vi "daqio_Upload_File.vi"(8 "error in (no error)":errorcluster, 10 "File to upload":T1={"File Type"="image", "label (File Name by default)"="", "File to be uploaded"=path ""}, 11 "daq.io type in":T2={"daq.io ref"=refnum, "daq.io API Base"="http://dashboard.daq.io/api/v1", "Device Key"="", "Account ID"="", "online"=TRUE, "SSL"=TRUE}) -> (0 "error out":errorcluster, 2 "asset ID":string, 3 "daq.io type out":T2={"daq.io ref"=refnum, "daq.io API Base"="http://dashboard.daq.io/api/v1", "Device Key"="", "Account ID"="", "online"=TRUE, "SSL"=TRUE})   [LabVIEW 2013, in "daqio minimal.lvlib"]
doc: "This VI uploads a new user file. It can be any file type. However, images and CSV files will be treated specially on daq.io, therefore make sure to select the correct file type, if you want features like the image preview to work. For PDF files, please select binary. \nThe VI will return the unique file ID that can be used to retrieve the file later and link it to a device."
uses:
  daqio minimal.lvlib
  _typedefs/daqio-Type.ctl
  <vilib>/httpClient/ClientHandle.ctl
  _typedefs/daqio-File.ctl
  _typedefs/daqio-File-Post.ctl
  <vilib>/httpClient/MultipartData.ctl
  _typedefs/daqio-Credentials-FGV.ctl
  <vilib>/Easy HTTP Client/Easy HTTP.lvlib
  <vilib>/httpClient/LabVIEWHTTPClient.lvlib
panel:
  out "JSON string":string
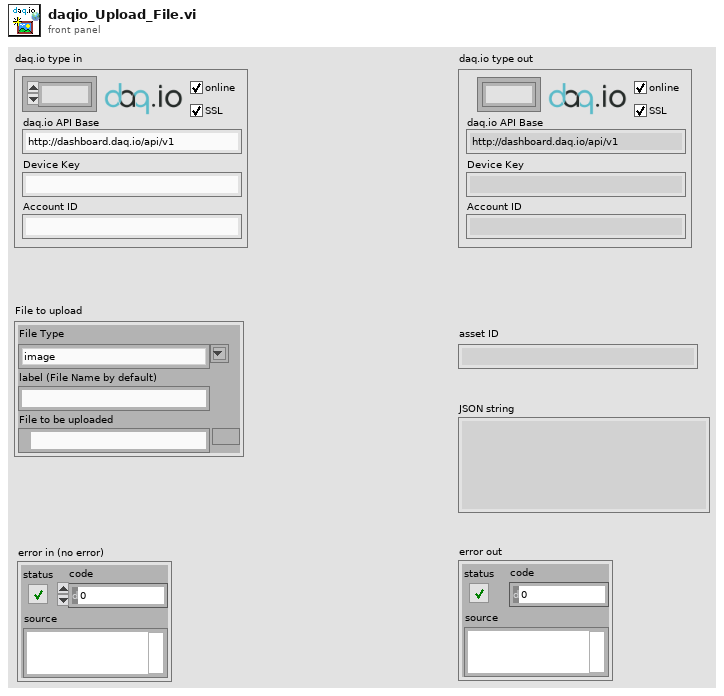
[diagram p1: front panel]
types:
  T1 = cluster{"File Type":string, "label (File Name by default)":string, "File to be uploaded":path}
  T2 = typedef "daqio minimal.lvlib/daqio-Type.ctl" = cluster{"daq.io ref":T3, "daq.io API Base":string, "Device Key":string, "Account ID":string, "online":bool, "SSL":bool}
  T3 = typedef "LabVIEWHTTPClient.lvlib/ClientHandle.ctl" = refnum<k1>
  T4 = typedef "daqio minimal.lvlib/daqio-Credentials-FGV.ctl" = enum16{"Generate", "Read"}
  T5 = typedef "LabVIEWHTTPClient.lvlib/MultipartData.ctl" = cluster{"Name":string, "Value":string, "File":path, "Filename":string, "MIME type":string}
  T6 = typedef "daqio minimal.lvlib/daqio-File-Post.ctl" = cluster{"file_type":string, "label":string, "original_file_name":string}
  T7 = typedef "daqio minimal.lvlib/daqio-File.ctl" = cluster{"id":string, "url":string, "file_type":string, "label":string, "original_file_name":string}
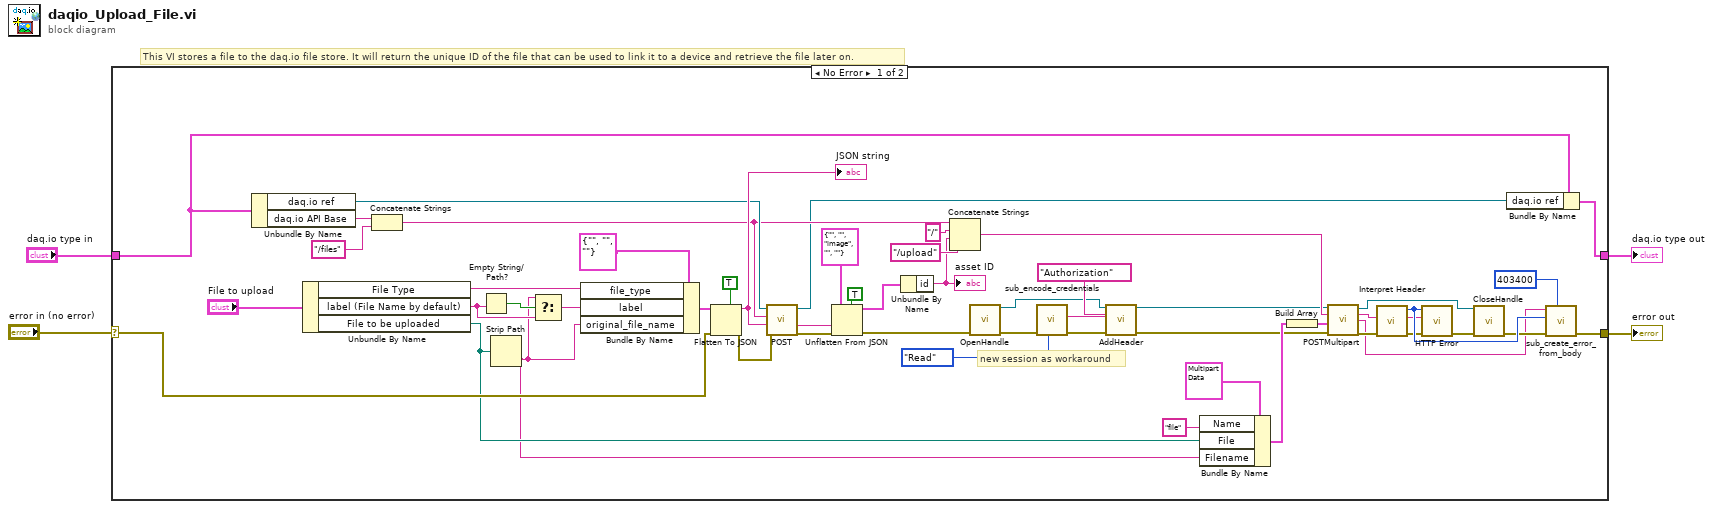
[diagram p0: block diagram]
diagram:
  # "This VI stores a file to the daq.io file store. It will return the unique ID of the file that can be used to link it to a device and retrieve the file later on."
  n1 = case shown="No Error" "error in (no error)" {
    selector: "error in (no error)" -> [w46 w58]
    tunnel: "daq.io type in" -> [w49 w59]
    tunnel: [w38 w59] -> w3
    tunnel: [w53 w58] -> w2
    frame No Error {
      # "new session as workaround"
      n2 = Unbundle By Name(w49) -> ("daq.io ref"=w44:T3, "daq.io API Base"=w52:string)
      n3 = Unbundle By Name("File to upload") -> ("File Type"=w22:string, "label (File Name by default)"=w47:string, "File to be uploaded"=w21:path)
      n4 = Concatenate Strings(w52, "/files") -> (w37:string)
      n5 = Empty String/Path?(string/path=w47) -> (empty?=w51:bool)
      n6 = Strip Path(path=w21) -> (name=w20:string)  [unwired: 1 out]
      n7 = Select(t=w20, s=w51, f=w47) -> (s? t:f=w50:string)
      n8 = Bundle By Name(cluster=T6 {"file_type"="", "label"="", "original_file_name"=""} ("Asset"), "file_type"=w22, "label"=w50, "original_file_name"=w20) -> (w56:T6)
      n9 = Flatten To JSON(enable LabVIEW extensions? (T)=TRUE, anything=w56, error in (no error)=w46) -> (JSON string=w55:string, 11:w57:errorcluster)
      "JSON string" <- w55
      n10 = call <vilib>:"POST.vi"("error in (no error)"=w57, "data"=w55, "url"=w37, "client handle"=w44) -> ("error out"=w41:errorcluster, "body"=w42:string, "client handle out"=w11:T3)  [unwired: 3 in, 2 out]
      n11 = Unflatten From JSON(enable LabVIEW extensions? (T)=TRUE, JSON string=w42, type and defaults=T7 {"id"="", "url"="", "file_type"="image", "label"="", "original_file_name"=""} ("Asset"), error in (no error)=w41) -> (value=w39:T7, error out=w17:errorcluster)  [unwired: 3 in]
      n12 = Unbundle By Name(w39) -> ("id"=w33:string)
      "asset ID" <- w33
      n13 = Concatenate Strings(w37, "/" ("string"), w33, "/upload" ("string")) -> (w31:string)
      n14 = call <vilib>:"OpenHandle.vi"("error in (no error)"=w17) -> ("client handle out"=w16:T3, "error out"=w13:errorcluster)  [unwired: 13 in]
      n15 = call "sub_encode_credentials.vi"("Command"=daqio-Credentials-FGV."Read", "error in"=w13) -> ("error out"=w12:errorcluster, "Stored Credentials"=w18:string)  [unwired: 7 in, 1 out]
      n16 = call <vilib>:"AddHeader.vi"("client handle"=w16, "header"="Authorization", "value"=w18, "error in (no error)"=w12) -> ("client handle out"=w15:T3, "error out"=w14:errorcluster)  [unwired: 10 in]
      n17 = Bundle By Name(cluster=T5 {"Name"="", "Value"="", "File"=path "", "Filename"="", "MIME type"="application/octet-stream"} ("Element"), "Name"="file", "File"=w21, "Filename"=w20) -> (w26:T5)
      n18 = Build Array(w26) -> (w25:T5[])
      n19 = call <vilib>:"POSTMultipart.vi"("client handle"=w15, "url"=w31, "data"=w25, "error in (no error)"=w14) -> ("client handle out"=w9:T3, "headers"=w28:string, "body"=w6:string, "error out"=w27:errorcluster)  [unwired: 8 in]
      n20 = call <vilib>:"Interpret Header.vi"("error in (no error)"=w27, "Header"=w28) -> ("error out"=w29:errorcluster, "HTTP Response"=w30:string, "HTTP Code"=w32:i32)  [unwired: 5 in, 2 out]
      n21 = call <vilib>:"HTTP Error.vi"("error in (no error)"=w29, "HTTP Response"=w30, "HTTP Code"=w32) -> ("error out"=w10:errorcluster)  [unwired: 8 in]
      n22 = call <vilib>:"CloseHandle.vi"("client handle"=w9, "error in (no error)"=w10) -> ("error out"=w8:errorcluster)  [unwired: 13 in]
      n23 = Bundle By Name(cluster=w49, "daq.io ref"=w11) -> (w38:T2)
      n24 = call "sub_create_error_from_body.vi"("error code"=403400, "error in (no error)"=w8, "http code"=w32, "body"=w6) -> ("error out"=w53:errorcluster)  [unwired: 7 in]
    }
    frame Error {
    }
  }
  "error out" <- w2
  "daq.io type out" <- w3
